vi "Format Variant into String Advance.vi"(6 "include Variant Attributes(F)":bool, 7 "Format String":string, 8 "error in (no error)":errorcluster, 11 "Variant":variant) -> (0 "error out":errorcluster, 2 "Type":T1, 3 "Data":string)   [LabVIEW 2017]
doc: "Formats any variant into a string, handling arrays, clusters, enums, refnums and LabVIEW classes. Set include Variant Attributes(F) to append the variant's attributes, and wire Format String to override the default formatting."
uses:
  <vilib>/Utility/Data Type/Type Definitions/Data Type.ctl
  <vilib>/Utility/Data Type/Type Definitions/Refnum Type.ctl
  <vilib>/Utility/Data Type/NI_Data Type.lvlib
  _openG/_reuse_openG.lvlib
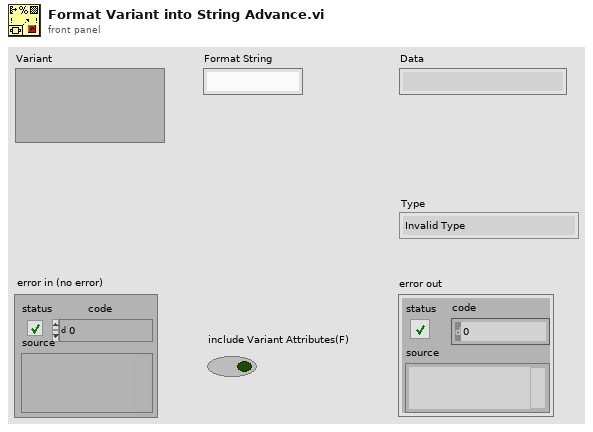
[diagram p1: front panel]
types:
  T1 = typedef "NI_Data Type.lvlib/Data Type.ctl" = enum8{"Invalid Type", "Void", "I8", "I16", "I32", "I64", "U8", "U16", "U32", "U64", "Single Float", "Double Float", "Extended Float", "Single Complex", "Double Complex", "Extended Complex", "Enum U8", "Enum U16", "Enum U32", "Enum U64", "Single Float With Unit", "Double Float With Unit", "Extended Float With Unit", "Single Complex with Unit", "Double Complex with Unit", "Extended Complex with Unit", "Boolean", "String", "Path", "Picture", "Tag", "Array", "Cluster", "Variant", "LV Variant", "Waveform", "Timestamp", "Digital Waveform", "Digital Data", "ExpressData", "Refnum", "External Data", "VI", "Poly VI", "LabVIEW Class Instance", "Fixed Point"}
  T2 = typedef "NI_Data Type.lvlib/Refnum Type.ctl" = enum16{"NotARefnum", "UnknownRefnum", "Generic", "Datalog", "ByteStream", "Device", "Occurence", "TCPNetConnection", "Auto", "Menu", "Imaq", "Hardware", "DataSocket", "Visa", "IVI", "UDPNetConnection", "Notifier", "Queue", "Irda", "EventReg", "DotNet", "UserEvent", "Callback", "UNUSED_EMPTY_POSITION", "BlueToothNetConnection", "LVObjApp", "LVObjVI", "LVObjUnknown", "GenericClass", "UserDefinedRefnumTag", "DataValue", "RT FIFO", "TDMS File"}
  T3 = cluster{"length":u16, "private":u8, "type":enum8{"<Null>", "I8", "I16", "I32", "I64", "U8", "U16", "U32", "U64", "SGL", "DBL", "EXT", "CSG", "CDB", "CXT", "0x0F", "0x10", "0x11", "0x12", "0x13", "0x14", "Enum U8", "Enum U16", "Enum U32", "Enum U64", "SGL PQ", "DBL PQ", "EXT PQ", "CSG PQ", "CDB PQ", "CXT PQ", "0x1F", "0x20", "Boolean", "0x22", "0x23", "0x24", "0x25", "0x26", "0x27", "0x28", "0x29", "0x2A", "0x2B", "0x2C", "0x2D", "0x2E", "0x2F", "String", "0x31", "Path", "Pict", "0x34", "0x35", "0x36", "DAQ", "0x38", "0x39", "0x3A", "0x3B", "0x3C", "0x3D", "0x3E", "0x3F", "Array", "0x41", "0x42", "0x43", "0x44", "0x45", "0x46", "0x47", "0x48", "0x49", "0x4A", "0x4B", "0x4C", "0x4D", "0x4E", "0x4F", "Cluster", "0x51", "0x52", "Variant", "Waveform", "0x55", "0x56", "0x57", "0x58", "0x59", "0x5A", "0x5B", "0x5C", "0x5D", "0x5E", "Fixed Point", "0x60", "0x61", "0x62", "0x63", "0x64", "0x65", "0x66", "0x67", "0x68", "0x69", "0x6A", "0x6B", "0x6C", "0x6D", "0x6E", "0x6F", "Refnum", "0x71", "0x72", "Set Collection", "Map Collection"}, "# elements":u16}
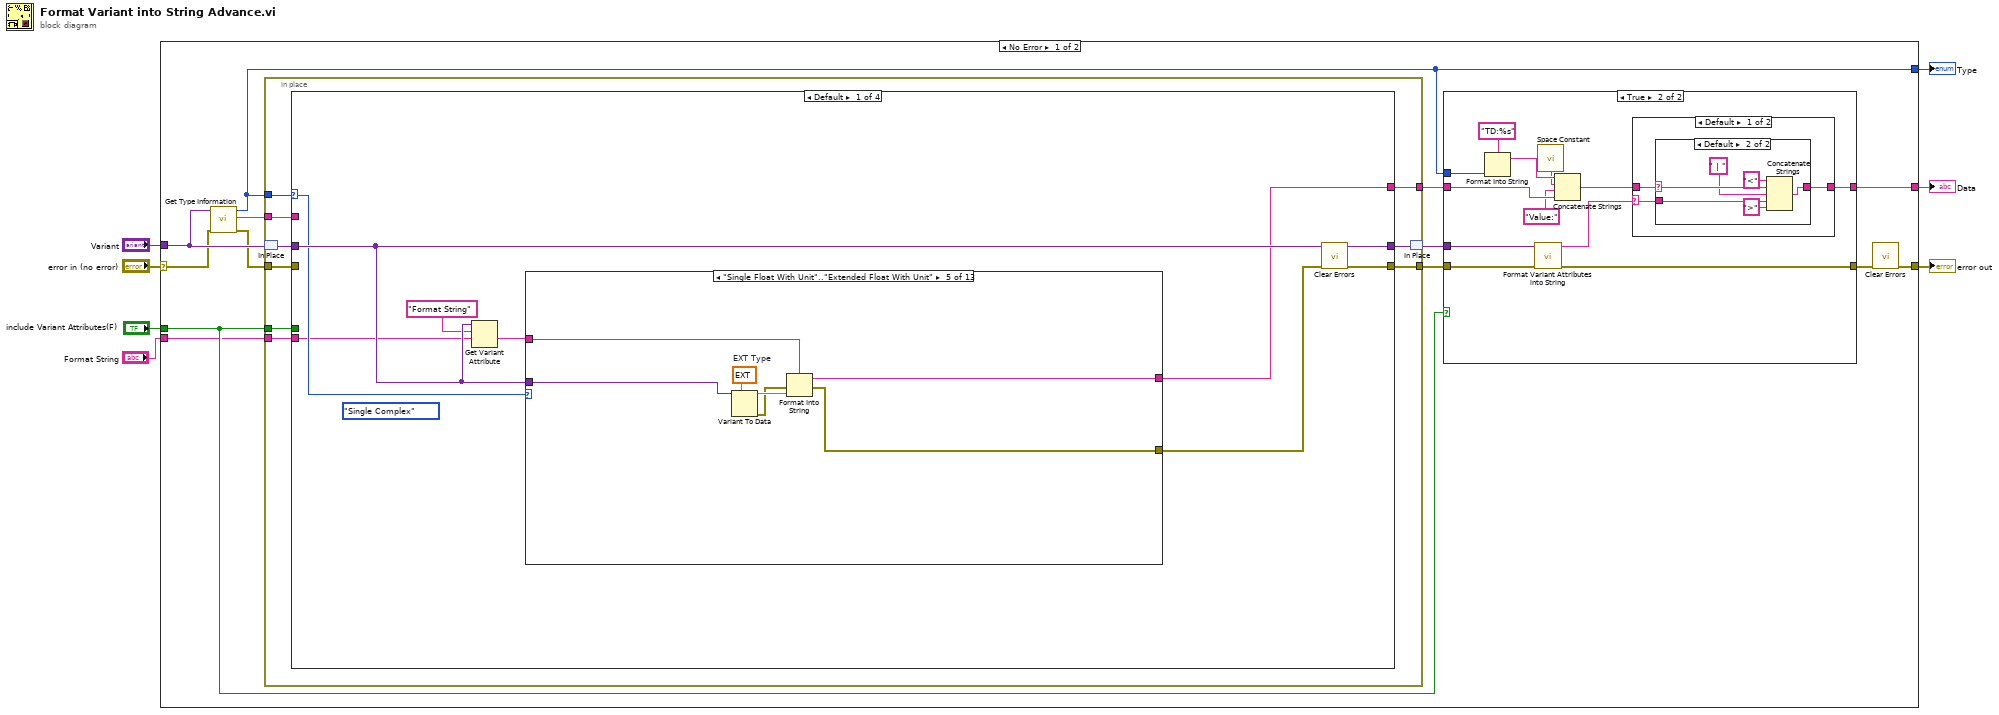
[diagram p0: block diagram]
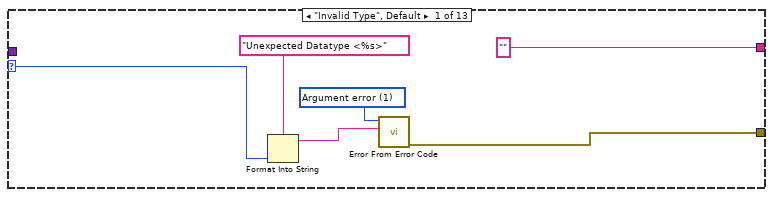
[diagram p5: hidden frame]
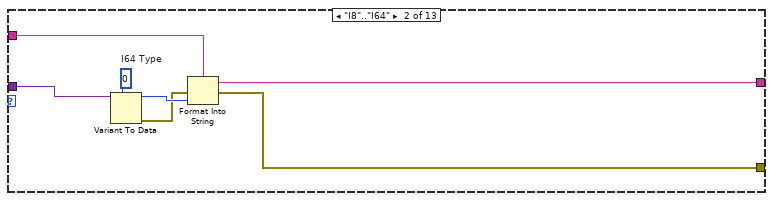
[diagram p6: hidden frame]
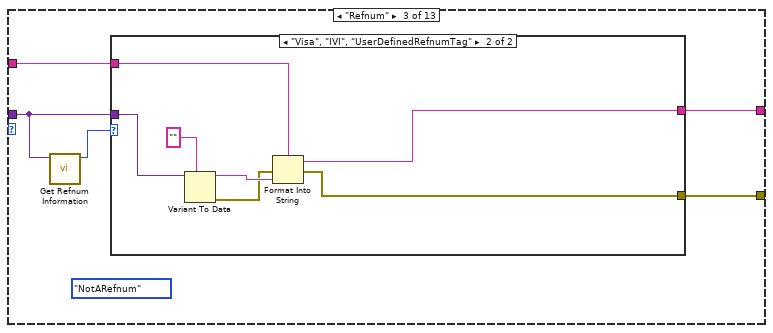
[diagram p7: hidden frame]
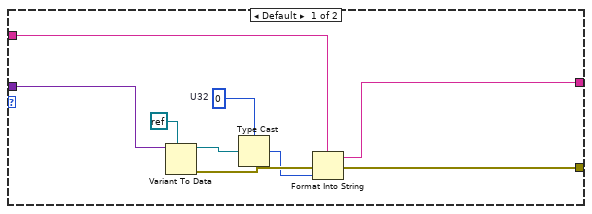
[diagram p8: hidden frame]
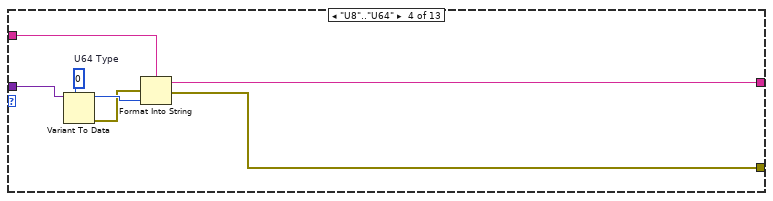
[diagram p9: hidden frame]
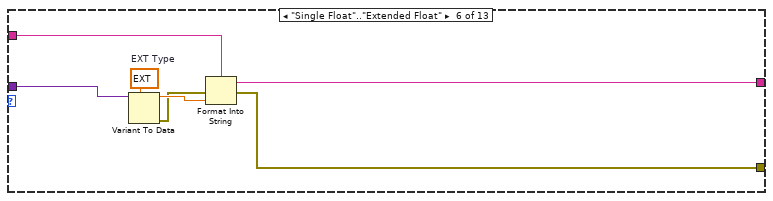
[diagram p10: hidden frame]
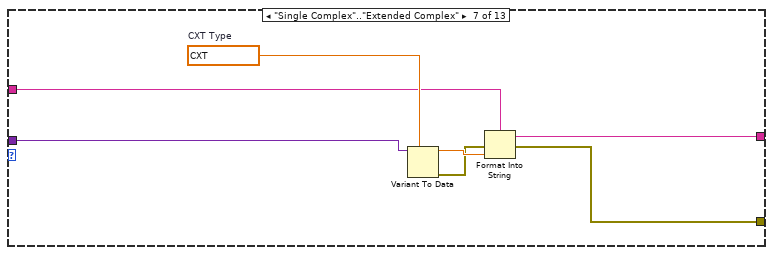
[diagram p11: hidden frame]
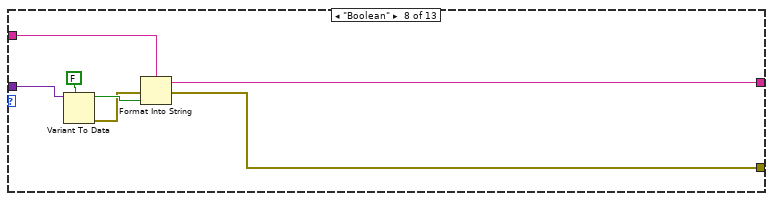
[diagram p12: hidden frame]
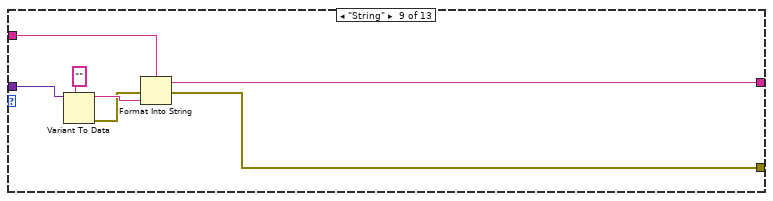
[diagram p13: hidden frame]
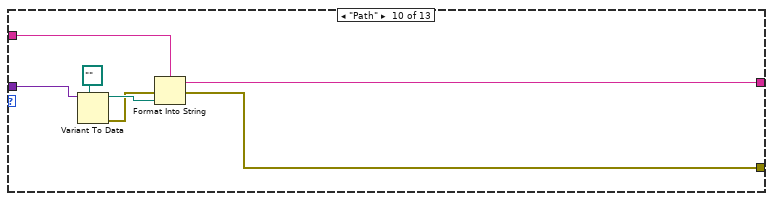
[diagram p14: hidden frame]
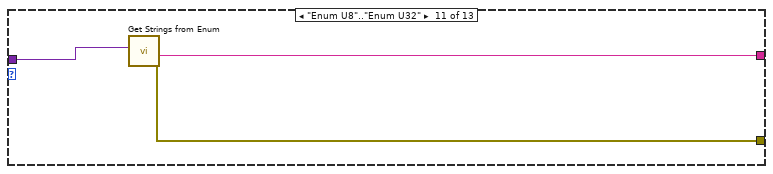
[diagram p15: hidden frame]
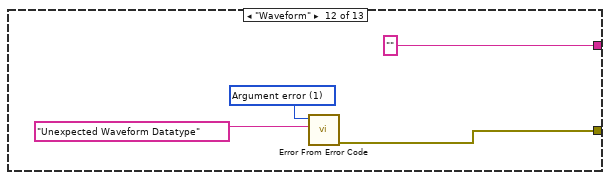
[diagram p16: hidden frame]
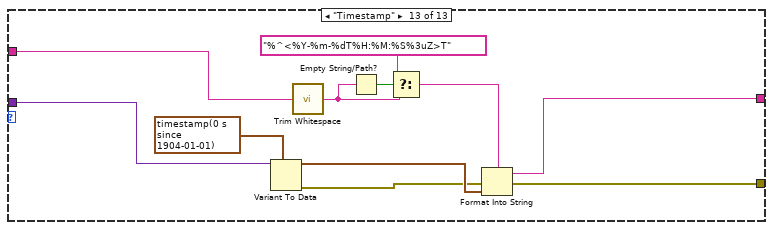
[diagram p17: hidden frame]
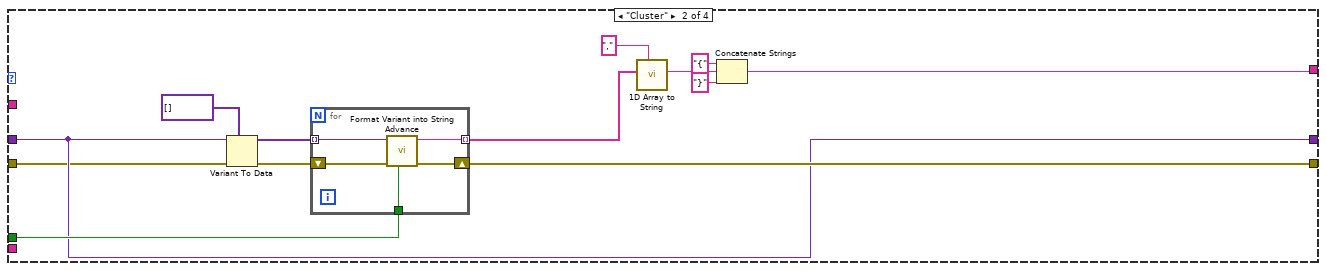
[diagram p18: hidden frame]
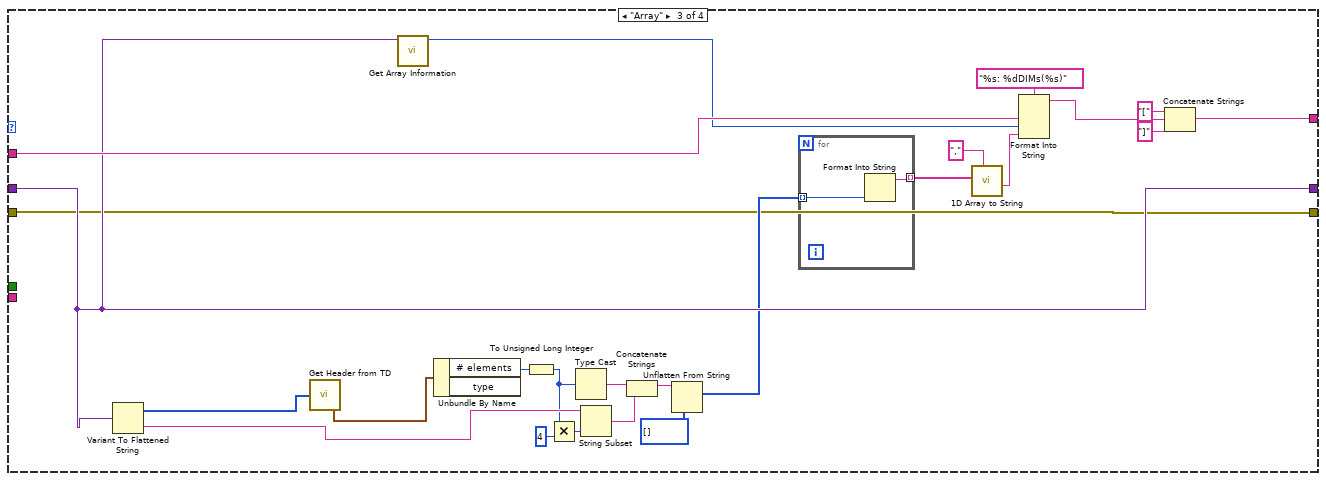
[diagram p19: hidden frame]
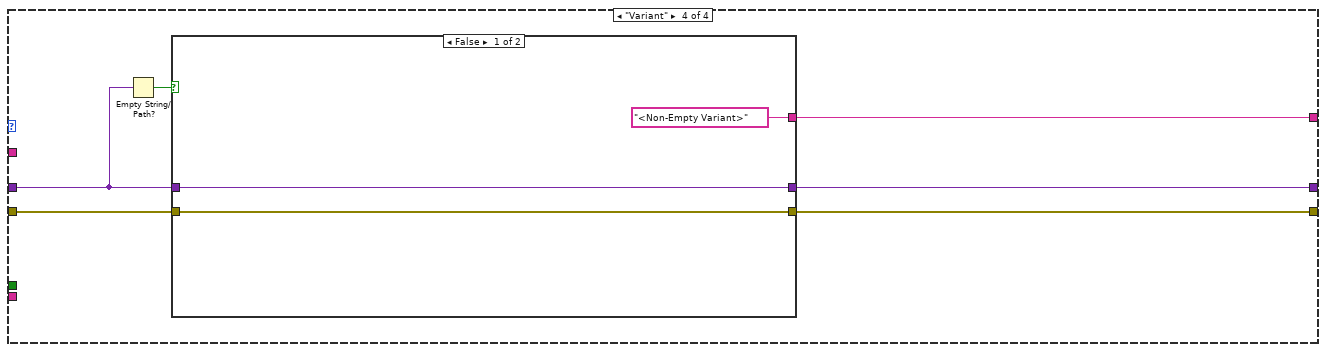
[diagram p20: hidden frame]
diagram:
  n1 = case shown="No Error" "error in (no error)" {
    selector: "error in (no error)" -> [w12 w221]
    tunnel: [w16 "!ERROR!" ("Output String")] -> w7
    tunnel: [w20 w221] -> w5
    tunnel: "Variant" -> [w13 _]
    tunnel: [w10 Data_Type."Invalid Type" ("Type")] -> w2
    tunnel: "include Variant Attributes(F)" -> [w14 _]
    tunnel: "Format String" -> [w8 _]
    frame No Error {
      n2 = call <vilib>:"Get Type Information.vi"("error in (no error)"=w12, "Variant"=w13) -> ("error out"=w11:errorcluster, "Name"=w9:string, "Type"=w10:T1)  [unwired: 5 in, 2 out]
      n3 = in-place {
        in-place-border: w11 -> [w54]
        in-place-border: w10 -> [w53]
        in-place-border: [w52] -> w19
        in-place-border: [w51] -> w17
        in-place-border: w14 -> [w48]
        in-place-border: w9 -> [w47]
        in-place-border: w8 -> [w46]
        n4 = in-place-match #1(w13) -> (w50:variant)
        n5 = case shown="Default" w53 {
          selector: w53 -> [w56 _ _ _]
          tunnel: [w59 w172 w204 w211] -> w51
          tunnel: [w60 w175 w183 w212] -> w52
          tunnel: w50 -> [w61 w167 w196 w208]
          tunnel: w54 -> [_ w164 w183 w213]
          tunnel: [w61 w167 w196 w209] -> w49
          tunnel: w48 -> [_ w169 _ _]
          tunnel: w47 -> [_ _ w197 _]
          tunnel: w46 -> [w55 _ _ _]
          frame Default {
            (unwired) Data_Type."Single Complex" ("Type")
            n6 = Get Variant Attribute(Variant=w61, name="Format String", default value (empty Variant)=w55) -> (value=w57:string)  [unwired: 1 in, 3 out]
            n7 = case shown="\"Single Float With Unit\"..\"Extended Float With Unit\"" w56 {
              selector: w56 -> [w64 _ _ _ _ _ _ _ _ _ _ _ _]
              tunnel: w61 -> [_ w74 w78 w102 w104 w111 w123 w131 w138 w145 w148 _ w163]
              tunnel: w57 -> [_ w72 w77 w100 w108 w115 w121 w125 w136 w143 _ _ w160]
              tunnel: ["" w71 w79 w99 w107 w114 w120 w129 w135 w142 w147 "" w161] -> w59
              tunnel: [w63 w69 w80 w97 w105 w112 w118 w126 w132 w139 w146 w152 w162] -> w62
              frame "Invalid Type", Default {
                w67 = 1 items=["No error", "Argument error", "Memory is full", "Out of zone", "End of file", "File already open", "Generic file I/O error", "File not found", "File permission error", "Disk is full", "Duplicate path", "Too many files open", "System feature not enabled", "Resource file not found", "Cannot add resource", "Resource not found", "Image not found", "Image memory error", "Pen does not exist", "Config type invalid", "Config token not found", "Config parse error", "Config memory error", "Bad external code format", "Bad external code offset", "External code not present", "Null window", "Destroy window error", "Null menu", "Print aborted", "Bad print record", "Print driver error", "Windows error during printing", "Memory error during printing", "Print dialog error", "Generic print error", "Invalid device refnum", "Device not found", "Device parameter error", "Device unit error", "Cannot open device", "Device call aborted", "Generic error", "Cancelled by user", "Object ID too low", "Object ID too high", "Object not in heap", "Unknown heap", "Unknown object (invalid DefProc)", "Unknown object (DefProc not in table)", "Message out of range", "Invalid (null) method", "Unknown message", "Manager call not supported", "Bad address", "Network operation in progress", "Network operation timed out", "Connection is busy", "Network attribute not supported", "Network error", "Address in use", "System out of memory", "Connection aborted", "Connection refused", "Not connected", "Already connected", "Connection closed", "Initialization error (interapplication manager)", "Bad occurrence", "Wait on unbound occurrence handler", "Occurrence queue overflow", "Datalog type conflict", "Unused", "Unrecognized type (interapplication manager)", "Memory corrupt", "Failed to make temporary DLL", "Old CIN version", "Drag socket not found", "Failed to load drop-object", "Failed to register OLE object", "Failed to release OLE object", "Format specifier type mismatch", "Unknown format specifier", "Too few format specifiers", "Too many format specifiers", "Scan failed", "Newer CIN version", "Error converting to variant", "Runtime menu error", "Password tampered", "Variant attribute not found", "Incompatible variant data type", "Event data is not available", "Event Store is not present", "Occurrence is not found", "Event Queue is not created", "Event info is not available", "Refnum passed is NULL", "Error retrieving Class GUID", "Error retrieving CoClass GUID", "Error retrieving TypeLib GUID.", "Bad built application magic bytes.", "Specific driver is different from the specific driver associated with the Logical Name.", "There is no session opened to the class driver.", "Max Error", "MAX - Error with config objects", "MAX - Error loading configuration", "MAX - Group not supported"]
                n8 = Format Into String(format string="Unexpected Datatype <%s>" ("Format String"), w64) -> (resulting string=w65:string)  [unwired: 2 in, 1 out]
                n9 = call "Error From Error Code.vi"("error message (\"\")"=w65, "error code (0)"=w67) -> ("error out"=w63:errorcluster)  [unwired: 7 in]
              }
              frame "I8".."I64" {
                w75 = i64 0  # I64 Type
                n10 = Variant To Data(type=w75, Variant=w74) -> (data=w73:i64, error out=w70:errorcluster)  [unwired: 1 in]
                n11 = Format Into String(format string=w72, error in=w70, w73) -> (resulting string=w71:string, error out=w69:errorcluster)  [unwired: 1 in]
              }
              frame "Refnum" {
                (unwired) Refnum_Type."NotARefnum" ("Reference Type")
                n12 = call <vilib>:"Get Refnum Information.vi"("Variant"=w78) -> ("Reference Type"=w76:T2)  [unwired: 7 in, 3 out]
                n13 = case shown="\"Visa\", \"IVI\", \"UserDefinedRefnumTag\"" w76 {
                  tunnel: [w81 w90] -> w80
                  tunnel: [w82 w93] -> w79
                  tunnel: w78 -> [w89 w91]
                  tunnel: w77 -> [w83 w92]
                  frame Default {
                    w86 = u32 0  # U32
                    n14 = Variant To Data(type=refnum<k0> refnum, Variant=w89) -> (data=w87:refnum<k0>, error out=w85:errorcluster)  [unwired: 1 in]
                    n15 = Type Cast(type=w86, x=w87) -> (*(type *) &x=w84:u32)
                    n16 = Format Into String(format string=w83, error in=w85, w84) -> (resulting string=w82:string, error out=w81:errorcluster)  [unwired: 1 in]
                  }
                  frame "Visa", "IVI", "UserDefinedRefnumTag" {
                    n17 = Variant To Data(type="" ("String Value"), Variant=w91) -> (data=w96:string, error out=w95:errorcluster)  [unwired: 1 in]
                    n18 = Format Into String(format string=w92, error in=w95, w96) -> (resulting string=w93:string, error out=w90:errorcluster)  [unwired: 1 in]
                  }
                }
              }
              frame "U8".."U64" {
                w103 = u64 0  # U64 Type
                n19 = Variant To Data(type=w103, Variant=w102) -> (data=w101:u64, error out=w98:errorcluster)  [unwired: 1 in]
                n20 = Format Into String(format string=w100, error in=w98, w101) -> (resulting string=w99:string, error out=w97:errorcluster)  [unwired: 1 in]
              }
              frame "Single Float With Unit".."Extended Float With Unit" {
                w110 = ext 0.0  # EXT Type
                n21 = Variant To Data(type=w110, Variant=w104) -> (data=w109:ext, error out=w106:errorcluster)  [unwired: 1 in]
                n22 = Format Into String(format string=w108, error in=w106, w109) -> (resulting string=w107:string, error out=w105:errorcluster)  [unwired: 1 in]
              }
              frame "Single Float".."Extended Float" {
                w117 = ext 0.0  # EXT Type
                n23 = Variant To Data(type=w117, Variant=w111) -> (data=w116:ext, error out=w113:errorcluster)  [unwired: 1 in]
                n24 = Format Into String(format string=w115, error in=w113, w116) -> (resulting string=w114:string, error out=w112:errorcluster)  [unwired: 1 in]
              }
              frame "Single Complex".."Extended Complex" {
                w124 = cxt 0.0+0.0i  # CXT Type
                n25 = Variant To Data(type=w124, Variant=w123) -> (data=w122:cxt, error out=w119:errorcluster)  [unwired: 1 in]
                n26 = Format Into String(format string=w121, error in=w119, w122) -> (resulting string=w120:string, error out=w118:errorcluster)  [unwired: 1 in]
              }
              frame "Boolean" {
                n27 = Variant To Data(type=FALSE, Variant=w131) -> (data=w130:bool, error out=w127:errorcluster)  [unwired: 1 in]
                n28 = Format Into String(format string=w125, error in=w127, w130) -> (resulting string=w129:string, error out=w126:errorcluster)  [unwired: 1 in]
              }
              frame "String" {
                n29 = Variant To Data(type="", Variant=w138) -> (data=w137:string, error out=w133:errorcluster)  [unwired: 1 in]
                n30 = Format Into String(format string=w136, error in=w133, w137) -> (resulting string=w135:string, error out=w132:errorcluster)  [unwired: 1 in]
              }
              frame "Path" {
                n31 = Variant To Data(type=path "", Variant=w145) -> (data=w144:path, error out=w140:errorcluster)  [unwired: 1 in]
                n32 = Format Into String(format string=w143, error in=w140, w144) -> (resulting string=w142:string, error out=w139:errorcluster)  [unwired: 1 in]
              }
              frame "Enum U8".."Enum U32" {
                n33 = call "Get Strings from Enum.vi"("Enum"=w148) -> ("error out"=w146:errorcluster, "String Value"=w147:string)  [unwired: 7 in, 2 out]
              }
              frame "Waveform" {
                w150 = 1 items=["No error", "Argument error", "Memory is full", "Out of zone", "End of file", "File already open", "Generic file I/O error", "File not found", "File permission error", "Disk is full", "Duplicate path", "Too many files open", "System feature not enabled", "Resource file not found", "Cannot add resource", "Resource not found", "Image not found", "Image memory error", "Pen does not exist", "Config type invalid", "Config token not found", "Config parse error", "Config memory error", "Bad external code format", "Bad external code offset", "External code not present", "Null window", "Destroy window error", "Null menu", "Print aborted", "Bad print record", "Print driver error", "Windows error during printing", "Memory error during printing", "Print dialog error", "Generic print error", "Invalid device refnum", "Device not found", "Device parameter error", "Device unit error", "Cannot open device", "Device call aborted", "Generic error", "Cancelled by user", "Object ID too low", "Object ID too high", "Object not in heap", "Unknown heap", "Unknown object (invalid DefProc)", "Unknown object (DefProc not in table)", "Message out of range", "Invalid (null) method", "Unknown message", "Manager call not supported", "Bad address", "Network operation in progress", "Network operation timed out", "Connection is busy", "Network attribute not supported", "Network error", "Address in use", "System out of memory", "Connection aborted", "Connection refused", "Not connected", "Already connected", "Connection closed", "Initialization error (interapplication manager)", "Bad occurrence", "Wait on unbound occurrence handler", "Occurrence queue overflow", "Datalog type conflict", "Unused", "Unrecognized type (interapplication manager)", "Memory corrupt", "Failed to make temporary DLL", "Old CIN version", "Drag socket not found", "Failed to load drop-object", "Failed to register OLE object", "Failed to release OLE object", "Format specifier type mismatch", "Unknown format specifier", "Too few format specifiers", "Too many format specifiers", "Scan failed", "Newer CIN version", "Error converting to variant", "Runtime menu error", "Password tampered", "Variant attribute not found", "Incompatible variant data type", "Event data is not available", "Event Store is not present", "Occurrence is not found", "Event Queue is not created", "Event info is not available", "Refnum passed is NULL", "Error retrieving Class GUID", "Error retrieving CoClass GUID", "Error retrieving TypeLib GUID.", "Bad built application magic bytes.", "Specific driver is different from the specific driver associated with the Logical Name.", "There is no session opened to the class driver.", "Max Error", "MAX - Error with config objects", "MAX - Error loading configuration", "MAX - Group not supported"]
                n34 = call "Error From Error Code.vi"("error message (\"\")"="Unexpected Waveform Datatype" ("Format String"), "error code (0)"=w150) -> ("error out"=w152:errorcluster)  [unwired: 7 in]
              }
              frame "Timestamp" {
                n35 = Variant To Data(type=timestamp(0 s since 1904-01-01) ("Time Stamp"), Variant=w163) -> (data=w158:timestamp, error out=w157:errorcluster)  [unwired: 1 in]
                n36 = call <vilib>:"Trim Whitespace.vi"("string"=w160) -> ("trimmed string"=w155:string)  [unwired: 1 in]
                n37 = Empty String/Path?(string/path=w155) -> (empty?=w153:bool)
                n38 = Select(t="%^<%Y-%m-%dT%H:%M:%S%3uZ>T" ("Format String"), s=w153, f=w155) -> (s? t:f=w156:string)
                n39 = Format Into String(format string=w156, error in=w157, w158) -> (resulting string=w161:string, error out=w162:errorcluster)  [unwired: 1 in]
              }
            }
            n40 = call <vilib>:"Clear Errors.vi"("error in (no error)"=w62) -> ("error out"=w60:errorcluster)  [unwired: 5 in, 1 out]
          }
          frame "Cluster" {
            n41 = Variant To Data(error in=w164, type=variant[] [] ("1D Array of Variants"), Variant=w167) -> (data=w166:variant[], error out=w165:errorcluster)
            n42 = for {
              tunnel: w166 -> [w181] mode=indexing
              tunnel: [w180] -> w176 mode=indexing
              shift-right: [w178] -> w175
              shift-left: w165 -> [w179]
              tunnel: w169 -> [w177]
              n43 = call "Format Variant into String Advance.vi"("include Variant Attributes(F)"=w177, "error in (no error)"=w179, "Variant"=w181) -> ("error out"=w178:errorcluster, "Data"=w180:string)  [unwired: 6 in, 1 out]
            }
            n44 = call "1D Array to String.vi"("delimiter (Tab)"=",", "Array of Strings"=w176) -> ("delimited string"=w174:string)  [unwired: 9 in]
            n45 = Concatenate Strings("{" ("string"), w174, "}" ("string")) -> (w172:string)
          }
          frame "Array" {
            n46 = Variant To Flattened String(Variant=w196) -> (data string=w193:string, 1:w182:i16[])
            n47 = call "Get Header from TD.vi"("Type Descriptor"=w182) -> ("Type Descriptor Header"=w192:T3)
            n48 = call <vilib>:"Get Array Information.vi"("Variant"=w196) -> ("Number of Dimensions"=w195:i32)  [unwired: 7 in, 3 out]
            n49 = Unbundle By Name(w192) -> ("# elements"=w191:u16)  [unwired: 1 out]
            n50 = To Unsigned Long Integer(number=w191) -> (unsigned 32bit integer=w184:u32)
            n51 = Multiply(x=w184, y=u32 4) -> (x*y=w188:u32)
            n52 = Type Cast(x=w184) -> (*(type *) &x=w185:string)  [unwired: 1 in]
            n53 = String Subset(string=w193, length (rest)=w188) -> (substring=w186:string)  [unwired: 1 in]
            n54 = Concatenate Strings(w185, w186) -> (w187:string)
            n55 = Unflatten From String(type=u32[] [] ("Size(s)"), binary string=w187) -> (value=w194:u32[])  [unwired: 3 in, 2 out]
            n56 = for {
              tunnel: w194 -> [w207] mode=indexing
              tunnel: [w206] -> w199 mode=indexing
              n57 = Format Into String(w207) -> (resulting string=w206:string)  [unwired: 3 in, 1 out]
            }
            n58 = call "1D Array to String.vi"("delimiter (Tab)"=",", "Array of Strings"=w199) -> ("delimited string"=w198:string)  [unwired: 9 in]
            n59 = Format Into String(format string="%s: %dDIMs(%s)", w197, w195, w198) -> (resulting string=w205:string)  [unwired: 2 in, 1 out]
            n60 = Concatenate Strings("[" ("string"), w205, "]" ("string")) -> (w204:string)
          }
          frame "Variant" {
            n61 = Empty String/Path?(string/path=w208) -> (empty?=w210:bool)
            n62 = case shown="False" w210 {
              tunnel: w213 -> [w215 w218]
              tunnel: [w215 w218] -> w212
              tunnel: ["<Non-Empty Variant>" ("Output String") _] -> w211
              tunnel: [w214 w217] -> w209
              tunnel: w208 -> [w214 w217]
              frame False {
              }
              frame True {
              }
            }
          }
        }
        n63 = in-place-match #1(w49) -> (w15:variant)
      }
      n64 = case shown="True" w14 {
        tunnel: w19 -> [w21 w34]
        tunnel: [w21 w33] -> w18
        tunnel: w17 -> [w22 w26]
        tunnel: [w22 w32] -> w16
        tunnel: w15 -> [_ w30]
        tunnel: w10 -> [_ w29]
        frame False {
        }
        frame True {
          n65 = Format Into String(format string="TD:%s", w29) -> (resulting string=w25:string)  [unwired: 2 in, 1 out]
          n66 = call "Format Variant Attributes into String.vi"("error in (no error)"=w34, "Variant"=w30) -> ("error out"=w33:errorcluster, "Data"=w31:string)  [unwired: 8 in]
          n67 = call <vilib>:"Space Constant.vi"() -> ("String"=w23:string)
          n68 = Concatenate Strings(w25, w23, "Value:" ("string"), w26) -> (w27:string)
          n69 = case shown="Default" w31 {
            selector: w31 -> [w35 _]
            tunnel: w27 -> [w37 w45]
            tunnel: [w36 w45] -> w32
            frame Default {
              n70 = case shown="Default" w37 {
                selector: w37 -> [_ w44]
                tunnel: [w38 w43] -> w36
                tunnel: w35 -> [w38 w42]
                frame "" {
                }
                frame Default {
                  n71 = Concatenate Strings("<" ("string"), w44, " | " ("string"), w42, ">" ("string")) -> (w43:string)
                }
              }
            }
            frame "" {
            }
          }
        }
      }
      n72 = call <vilib>:"Clear Errors.vi"("error in (no error)"=w18) -> ("error out"=w20:errorcluster)  [unwired: 5 in, 1 out]
    }
    frame Error {
    }
  }
  "Data" <- w7
  "error out" <- w5
  "Type" <- w2
